vi "Dump Switch Readback test.vi"() -> (0 "Dump Switch Readback OK":bool)   [LabVIEW 2015]
uses:
  <vilib>/DAQmx/read.llb/DAQmx Read (Digital Bool 1Line 1Point).vi
  <vilib>/DAQmx/write.llb/DAQmx Write (Digital Bool 1Line 1Point).vi
  <vilib>/DAQmx/miscellaneous.llb/DAQmx Fill In Error Info.vi
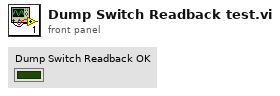
[diagram p1: front panel]
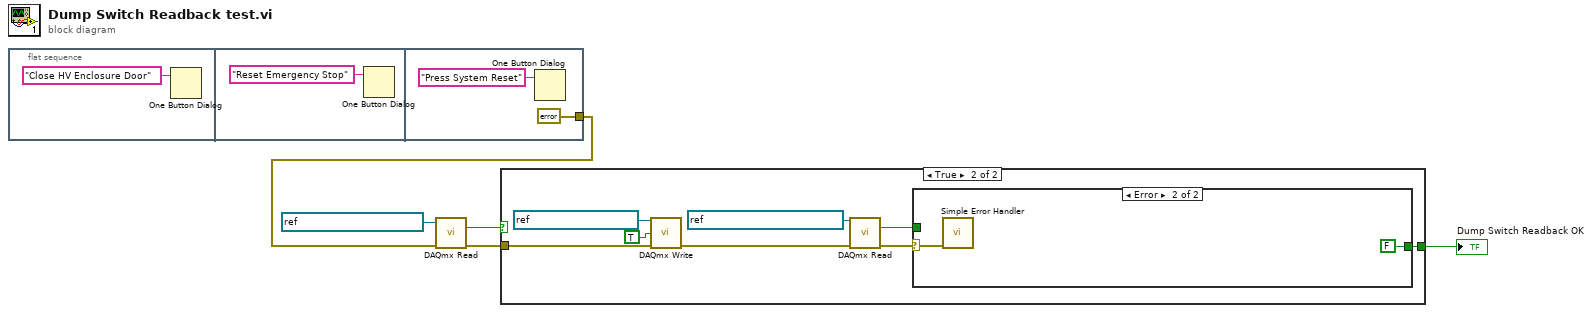
[diagram p0: block diagram]
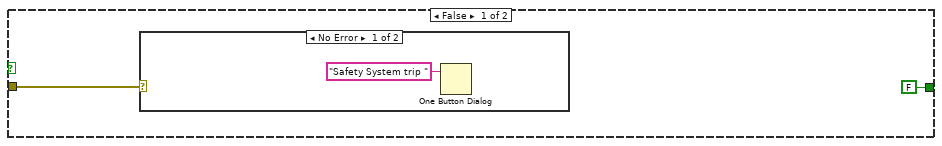
[diagram p2: hidden frame]
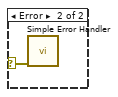
[diagram p3: hidden frame]
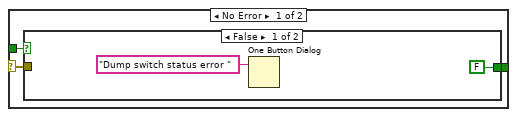
[diagram p4: hidden frame]
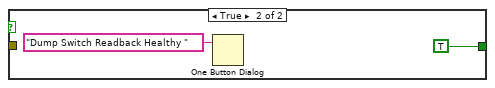
[diagram p5: hidden frame]
diagram:
  n1 = flat-sequence {
    tunnel: [errorcluster {"status"=FALSE, "code"=0, "source"=""} ("error constant")] -> w5
    frame #0 {
      n2 = One Button Dialog(message="Close HV Enclosure Door") -> ()  [unwired: 1 in, 1 out]
    }
    frame #1 {
      n3 = One Button Dialog(message="Reset Emergency Stop") -> ()  [unwired: 1 in, 1 out]
    }
    frame #2 {
      n4 = One Button Dialog(message="Press System Reset") -> ()  [unwired: 1 in, 1 out]
    }
  }
  n5 = call-poly <vilib>:"DAQmx Read.vi"("task/channels in"=refnum<k21> "DI1 Safety System trip" ("DAQmx Global Channel"), "error in"=w5) -> ("data"=w3:bool, "error out"=w4:errorcluster)  [unwired: 11 in, 1 out]
  n6 = case shown="True" w3 {
    tunnel: w4 -> [w11 w19]
    tunnel: [FALSE w14] -> w1
    frame False {
      n7 = case shown="No Error" w11 {
        selector: w11 -> [_ w13]
        frame No Error {
          n8 = One Button Dialog(message="Safety System trip ") -> ()  [unwired: 1 in, 1 out]
        }
        frame Error {
          n9 = call <vilib>:"Simple Error Handler.vi"("error in (no error)"=w13) -> ()  [unwired: 4 in, 5 out]
        }
      }
    }
    frame True {
      n10 = call-poly <vilib>:"DAQmx Write.vi"("task/channels in"=refnum<k21> "DO4 Dump Switch" ("DAQmx Global Channel"), "data"=TRUE, "error in"=w19) -> ("error out"=w18:errorcluster)  [unwired: 10 in, 2 out]
      n11 = call-poly <vilib>:"DAQmx Read.vi"("task/channels in"=refnum<k21> "DI5 Dump Switch mimic" ("DAQmx Global Channel"), "error in"=w18) -> ("data"=w16:bool, "error out"=w15:errorcluster)  [unwired: 11 in, 1 out]
      n12 = case shown="Error" w15 {
        selector: w15 -> [w23 w30]
        tunnel: w16 -> [w24 _]
        tunnel: [w22 FALSE] -> w14
        frame No Error {
          n13 = case shown="False" w24 {
            tunnel: w23 -> [_ _]
            tunnel: [FALSE TRUE] -> w22
            frame False {
              n14 = One Button Dialog(message="Dump switch status error ") -> ()  [unwired: 1 in, 1 out]
            }
            frame True {
              n15 = One Button Dialog(message="Dump Switch Readback Healthy ") -> ()  [unwired: 1 in, 1 out]
            }
          }
        }
        frame Error {
          n16 = call <vilib>:"Simple Error Handler.vi"("error in (no error)"=w30) -> ()  [unwired: 4 in, 5 out]
        }
      }
    }
  }
  "Dump Switch Readback OK" <- w1
